vi "Fault_ID_Parse.vi"(8 "Enum":enum16{"Sequence", "Table"}(ring), 11 "Numeric":u32) -> (3 "String":string)   [LabVIEW 2021]
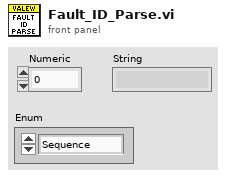
[diagram p1: front panel]
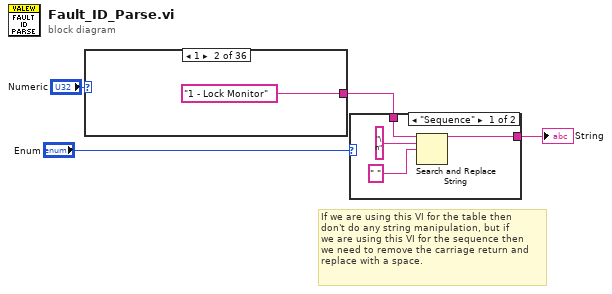
[diagram p0: block diagram]
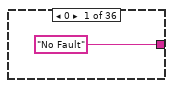
[diagram p3: hidden frame]
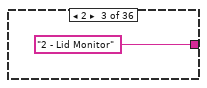
[diagram p4: hidden frame]
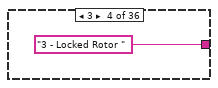
[diagram p5: hidden frame]
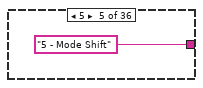
[diagram p6: hidden frame]
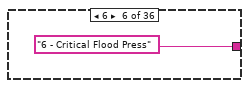
[diagram p7: hidden frame]
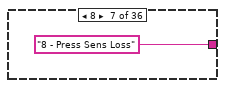
[diagram p8: hidden frame]
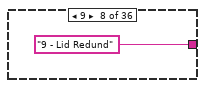
[diagram p9: hidden frame]
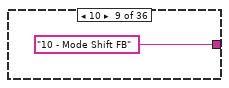
[diagram p10: hidden frame]
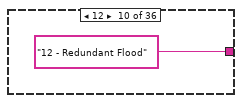
[diagram p11: hidden frame]
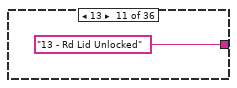
[diagram p12: hidden frame]
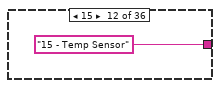
[diagram p13: hidden frame]
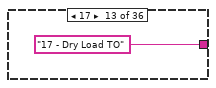
[diagram p14: hidden frame]
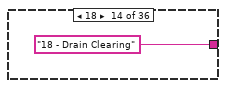
[diagram p15: hidden frame]
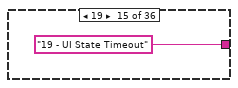
[diagram p16: hidden frame]
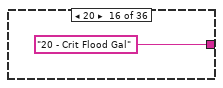
[diagram p17: hidden frame]
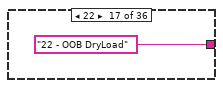
[diagram p18: hidden frame]
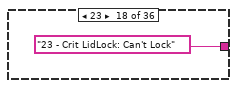
[diagram p19: hidden frame]
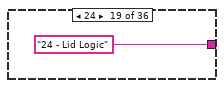
[diagram p20: hidden frame]
diagram:
  # "If we are using this VI for the table then\ndon't do any string manipulation, but if\nwe are using this VI for the sequence then\nwe need to remove the carriage return and\nreplace with a space."
  n1 = case shown="1" "Numeric" {
    selector: "Numeric" -> [_ _ _ _ _ _ _ _ _ _ _ _ _ _ _ _ _ _ _ _ _ _ _ _ _ _ _ _ _ _ _ _ _ _ _ w41]
    tunnel: ["No Fault" "1 - Lock Monitor" "2 - Lid Monitor" "3 - Locked Rotor " "5 - Mode Shift" "6 - Critical Flood Press" "8 - Press Sens Loss" "9 - Lid Redund" "10 - Mode Shift FB" "12 - Redundant Flood" "13 - Rd Lid Unlocked" "15 - Temp Sensor" "17 - Dry Load TO" "18 - Drain Clearing" "19 - UI State Timeout" "20 - Crit Flood Gal" "22 - OOB DryLoad" "23 - Crit LidLock: Can't Lock" "24 - Lid Logic" "25 - Press Sens Dropout" "26 - OOB Redist" "27 - Water Access" "28 - ADC Knob" "29 - Suds Lock" "30 - Stuck Button" "31 - OOB Fallback" "32 - Crit LidLock: Can't Unlock" "100 - Accelrmtr Comm" "101 - Flood Warning" "102 - Clock Mon" "103 - LidLock Failure" "104 - Adaptive Drain" "105 - Flood Warn Gal" "106 - Target Spin Speed Timeout" "107 - Target Spin Speed Dropout" w40] -> w3
    frame 0 {
    }
    frame 1 {
    }
    frame 2 {
    }
    frame 3 {
    }
    frame 5 {
    }
    frame 6 {
    }
    frame 8 {
    }
    frame 9 {
    }
    frame 10 {
    }
    frame 12 {
    }
    frame 13 {
    }
    frame 15 {
    }
    frame 17 {
    }
    frame 18 {
    }
    frame 19 {
    }
    frame 20 {
    }
    frame 22 {
    }
    frame 23 {
    }
    frame 24 {
    }
    frame 25 {
    }
    frame 26 {
    }
    frame 27 {
    }
    frame 28 {
    }
    frame 29 {
    }
    frame 30 {
    }
    frame 31 {
    }
    frame 32 {
    }
    frame 100 {
    }
    frame 101 {
    }
    frame 102 {
    }
    frame 103 {
    }
    frame 104 {
    }
    frame 105 {
    }
    frame 106 {
    }
    frame 107 {
    }
    frame Default {
      n2 = Number To Decimal String(number=w41) -> (decimal integer string=w40:string)  [unwired: 1 in]
    }
  }
  n3 = case shown="\"Sequence\"" "Enum" {
    tunnel: w3 -> [w45 w46]
    tunnel: [w42 w46] -> w2
    frame "Sequence" {
      n4 = Search and Replace String(input string=w45, search string="\n", replace string=" " ("replace string (\"\")")) -> (result string=w42:string)  [unwired: 5 in, 3 out]
    }
    frame "Table" {
    }
  }
  "String" <- w2
